vi "HW_GEN - Search for Modu CFG according to Tag.vi"(10 "ModuTag":string, 11 "ModuCFG[]":T1[](array[typedef])) -> (2 "find?":bool, 3 "ModuCFG out":T1, 5 "idx":i32)   [LabVIEW 2016]
uses:
  Ctrls/HardWare _ Module Configuration.ctl
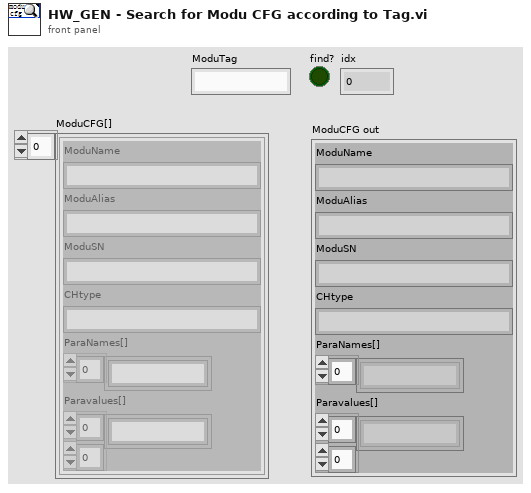
[diagram p1: front panel]
types:
  T1 = typedef "HardWare _ Module Configuration.ctl" = cluster{"ModuName":string, "ModuAlias":string, "ModuSN":string, "CHtype":string, "ParaNames[]":string[], "Paravalues[]":string[][]}
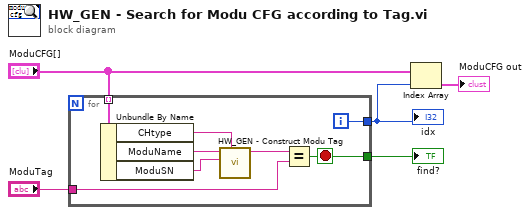
[diagram p0: block diagram]
diagram:
  n1 = for {
    tunnel: "ModuTag" -> [w13]
    tunnel: [w12] -> w4
    tunnel: "ModuCFG[]" -> [w11] mode=indexing
    tunnel: [w10] -> w2
    i -> [w10]
    stop <- w12 stop-if-true
    n2 = Unbundle By Name(w11) -> ("CHtype"=w9:string, "ModuName"=w8:string, "ModuSN"=w7:string)
    n3 = call "HW_GEN - Construct Modu Tag.vi"("ChanType"=w9, "ModSN"=w7, "ModName"=w8) -> ("String"=w6:string)  [unwired: 8 in]
    n4 = Equal?(x=w6, y=w13) -> (x = y?=w12:bool)
  }
  "find?" <- w4
  "idx" <- w2
  n5 = Index Array(array="ModuCFG[]", index=w2) -> (element=→"ModuCFG out":T1)
